vi "Configure Event Search (Serial Bus - Flexray).vi"(5 "Cycle Value (-1)":i32=-1, 6 "Frame ID (0)":i32, 7 "Data Length (1)":i32=1, 8 "error in (no error)":errorcluster, 9 "Data (0xXX)":string="0xXX", 10 "Search Operation (0: Frame)":i32(ring) items=["Frame", "Cycle", "Data", "Header CRC Error", "Frame CRC Error", "All Errors"], 11 "VISA resource name":refnum<visa-resource-name>) -> (0 "error out":errorcluster, 3 "VISA resource name out":refnum<visa-resource-name>)   [LabVIEW 2010, in "Agilent 2000 3000 X-Series.lvlib"]
doc: "Configures the event search of FlexRay bus."
uses:
  <instrlib>/Agilent 2000 3000 X-Series/Agilent 2000 3000 X-Series.lvlib
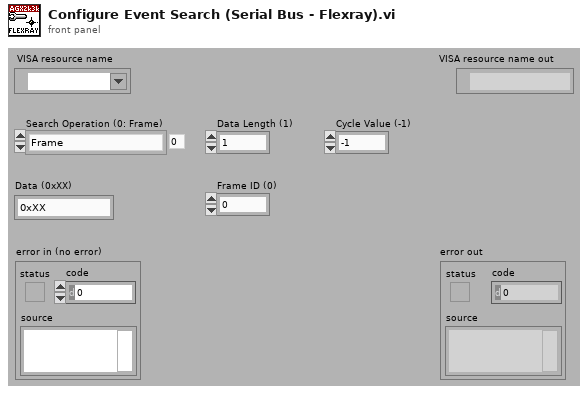
[diagram p1: front panel]
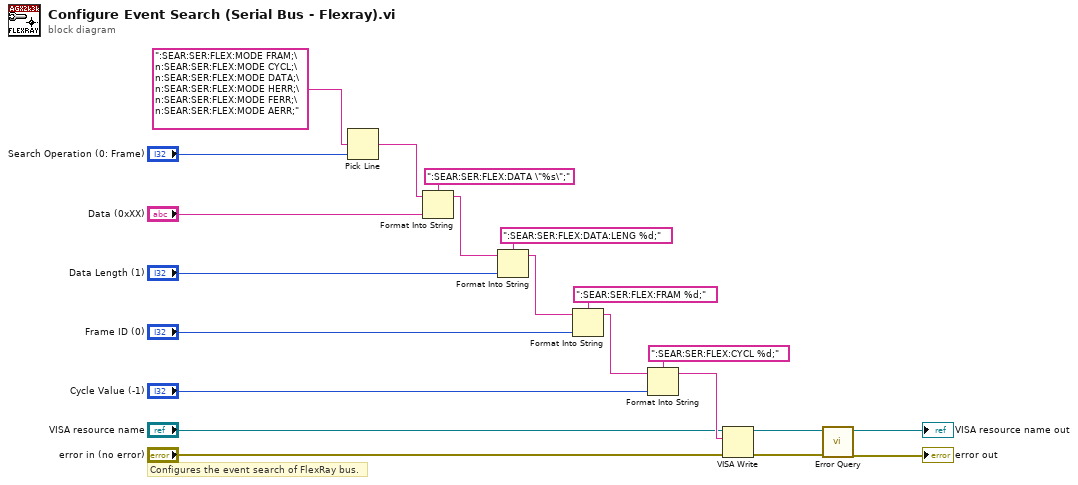
[diagram p0: block diagram]
diagram:
  # "Configures the event search of FlexRay bus."
  n1 = Pick Line(multi-line string=":SEAR:SER:FLEX:MODE FRAM;\n:SEAR:SER:FLEX:MODE CYCL;\n:SEAR:SER:FLEX:MODE DATA;\n:SEAR:SER:FLEX:MODE HERR;\n:SEAR:SER:FLEX:MODE FERR;\n:SEAR:SER:FLEX:MODE AERR;", line index="Search Operation (0: Frame)") -> (output string=w19:string)  [unwired: 1 out]
  n2 = Format Into String(format string=":SEAR:SER:FLEX:DATA \"%s\";", initial string=w19, "Data (0xXX)") -> (resulting string=w16:string)  [unwired: 1 in, 1 out]
  n3 = Format Into String(format string=":SEAR:SER:FLEX:DATA:LENG %d;", initial string=w16, "Data Length (1)") -> (resulting string=w13:string)  [unwired: 1 in, 1 out]
  n4 = Format Into String(format string=":SEAR:SER:FLEX:FRAM %d;", initial string=w13, "Frame ID (0)") -> (resulting string=w10:string)  [unwired: 1 in, 1 out]
  n5 = Format Into String(format string=":SEAR:SER:FLEX:CYCL %d;", initial string=w10, "Cycle Value (-1)") -> (resulting string=w7:string)  [unwired: 1 in, 1 out]
  n6 = VISA Write(VISA resource name="VISA resource name", write buffer=w7, error in (no error)="error in (no error)") -> (VISA resource name out=w4:refnum<visa-resource-name>, error out=w3:errorcluster)  [unwired: 1 out]
  n7 = call <instrlib>:"Error Query.vi"("error in (no error)"=w3, "VISA resource name"=w4) -> ("error out"=→"error out":errorcluster, "VISA resource name out"=→"VISA resource name out":refnum<visa-resource-name>)  [unwired: 8 out]
